vi "Measurement_Loop.vi"() -> ()   [LabVIEW 2011]
panel:
  out "Reading\nPoint":i32=4
  in  "Read Next Point":bool
  in  "stop":bool
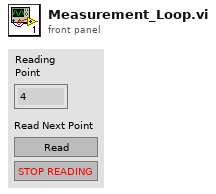
[diagram p1: front panel]
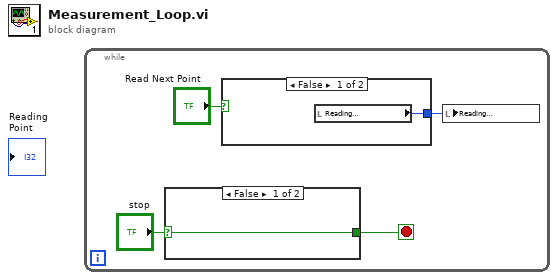
[diagram p0: block diagram]
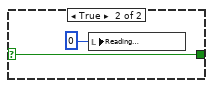
[diagram p2: hidden frame]
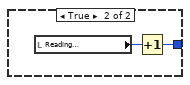
[diagram p3: hidden frame]
diagram:
  n1 = while {
    stop <- w1 stop-if-true
    n2 = case shown="False" "stop" {
      selector: "stop" -> [w5 w6]
      tunnel: [w5 w6] -> w1
      frame False {
      }
      frame True {
        n3 = local write "Reading\nPoint"(0) -> ()
      }
    }
    n4 = case shown="False" "Read Next Point" {
      tunnel: [w8 w10] -> w4
      frame False {
        n5 = local read "Reading\nPoint"() -> (w8:i32)
      }
      frame True {
        n6 = local read "Reading\nPoint"() -> (w9:i32)
        n7 = Increment(x=w9) -> (x+1=w10:i32)
      }
    }
    n8 = local write "Reading\nPoint"(w4) -> ()
  }
